vi "Program_VLIW_array.vi"(0 "path in":path=path "C:/Program Files/SpinCore/SpinAPI/dll/spinapi.dll", 1 "board_num":i32, 2 "PulseBlaster\nVLIW Array":T1(array[cluster])=[{"Output Bits"=4739583, "Data Field"=0, "OP Code"=1, "Delay Count"=99999999997}] {"OP Code" format="%.0x"; "Output Bits" format="%x"}, 3 "error in":errorcluster) -> (5 "path out":path, 7 "error out":errorcluster)   [LabVIEW 2013, in "SpinAPI-Interface.lvlib"]
doc: "PBcard_load: \nThis vi \n1) resets the PB, (consists of 4 steps)\n2) writes an array of VLIW's (very long instruction word) to the PB memory\n3) sends \"program finished\".\nAfter completion, a \"start\" command to the PB will make it run the programmed sequence. \n\nThe VLIW is implemented as a cluster of four integers (24bit, 20bit, 4bit, 32bit).\n\nNOTE: NO ERROR CHECKING IS PERFORMED. Error checking is supposedly taken care of before the VLIW array image is made, for example by Add_VLIW, which writes a PulseBlaster command to an array in memory. An"
uses:
  SpinAPI-Interface.lvlib
panel:
  # "(24 bits)"
  # "(20 bits)"
  # "(4 bits)"
  # "(32 bits)"
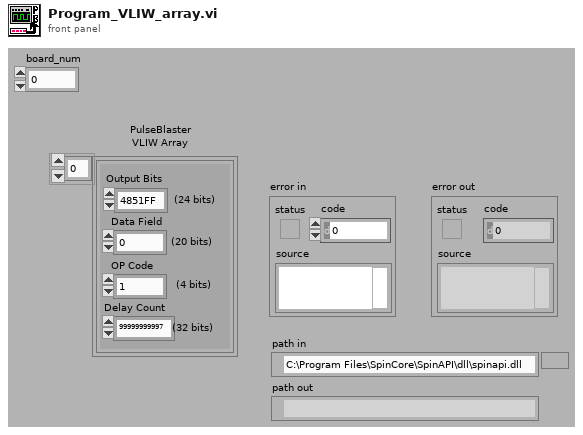
[diagram p1: front panel]
types:
  T1 = cluster{"Output Bits":u32, "Data Field":u32, "OP Code":u8, "Delay Count":u64}[]
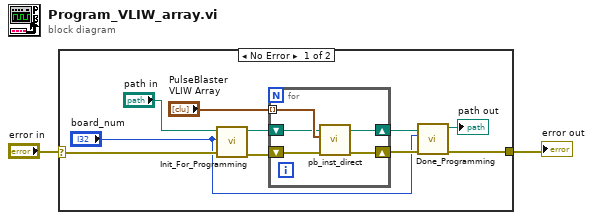
[diagram p0: block diagram]
diagram:
  n1 = case shown="No Error" "error in" {
    selector: "error in" -> [w12 w18]
    tunnel: [w9 w18] -> w1
    frame No Error {
      n2 = call "Init_For_Programming.vi"("error in (no error)"=w12, "board_num"="board_num", "path in"="path in") -> ("error out"=w11:errorcluster, "path out"=w7:path)  [unwired: 7 in]
      n3 = for {
        tunnel: "PulseBlaster\nVLIW Array" -> [w16] mode=indexing
        shift-right: [w13] -> w10
        shift-left: w11 -> [w17]
        shift-right: [w14] -> w6
        shift-left: w7 -> [w15]
        n4 = call "pb_inst_direct.vi"("error in (no error)"=w17, "PulseBlaster\nVLIW"=w16, "path in"=w15) -> ("error out"=w13:errorcluster, "path out"=w14:path)  [unwired: 7 in]
      }
      n5 = call "Done_Programming.vi"("error in (no error)"=w10, "board_num"="board_num", "path in"=w6) -> ("error out"=w9:errorcluster, "path out"=→"path out":path)  [unwired: 7 in]
    }
    frame Error {
    }
  }
  "error out" <- w1
